vi "minimax.vi"(0 "depth":i32=-1, 1 "redTurn":i32=-1, 2 "mode/difficulty":i32, 5 "mX":i32=-1, 7 "mY":i32=-1, 9 "exist":i32[][](array[numeric])=[[0, 0, 0, 0, 0, 0, 0, 0], [0, 0, 0, 0, 0, 0, 0, 0], [0, 0, 0, 0, 0, 0, 0, 0], [0, 0, 0, 0, 0, 0, 0, 0], [0, 0, 0, 0, 0, 0, 0, 0], [0, 0, 0, 0, 0, 0, 0, 0], [0, 0, 0, 0, 0, 0, 0, 0], [0, 0, 0, 0, 0, 0, 0, 0]], 11 "pos":i32[][](array[numeric])=[[0, 0, 0, 0, 0, 0, 0, 0], [0, 0, 0, 0, 0, 0, 0, 0], [0, 0, 0, 0, 0, 0, 0, 0], [0, 0, 0, 0, 0, 0, 0, 0], [0, 0, 0, 0, 0, 0, 0, 0], [0, 0, 0, 0, 0, 0, 0, 0], [0, 0, 0, 0, 0, 0, 0, 0], [0, 0, 0, 0, 0, 0, 0, 0]], 12 "alpha":i32=-1, 13 "beta":i32=-1) -> (4 "minimax":dbl, 6 "mXnew":i32=-1, 8 "mYnew":i32=-1, 10 "existNew":i32[][](array[numeric]), 15 "posNew":i32[][](array[numeric]))   [LabVIEW 2022 SP3, in "subvis.lvlib"]
uses:
  subvis.lvlib
panel:
  out "j":i32
  out "i":i32
  out "h":dbl
  out "newS.exist":i32[][](array[numeric])
  out "newS.pos":i32[][](array[numeric])
  out "newAvailables":i32[][](array[numeric])
  out "finish":bool
  out "bestHeu":dbl
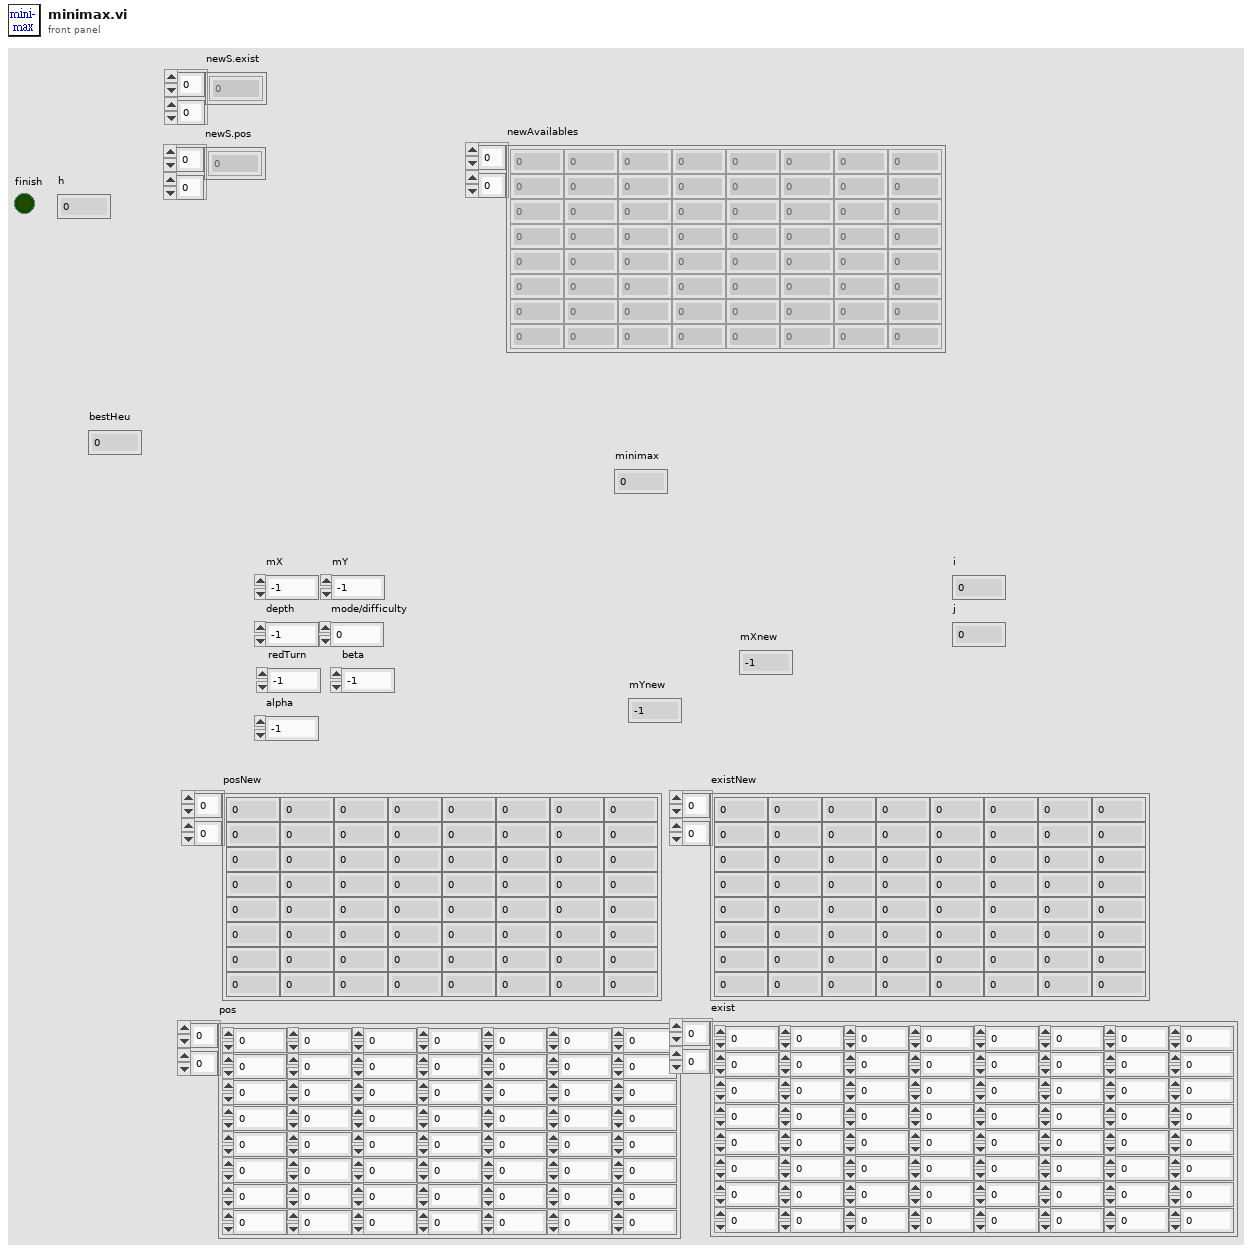
[diagram p1: front panel]
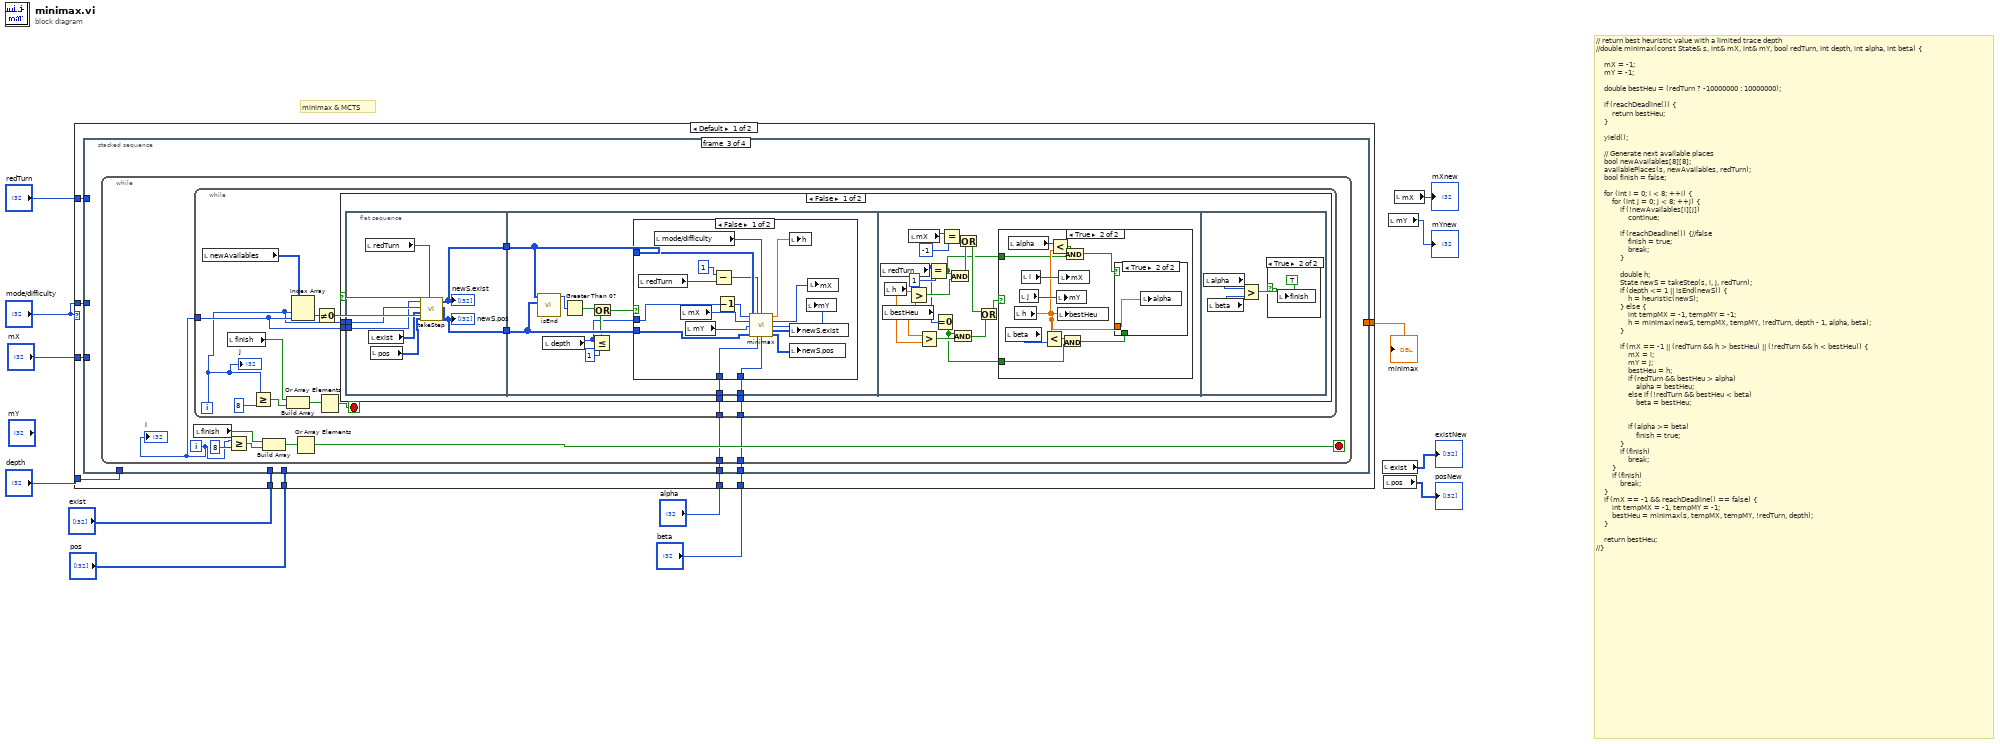
[diagram p0: block diagram]
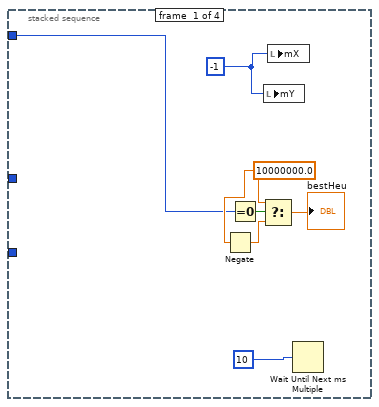
[diagram p2: hidden frame]
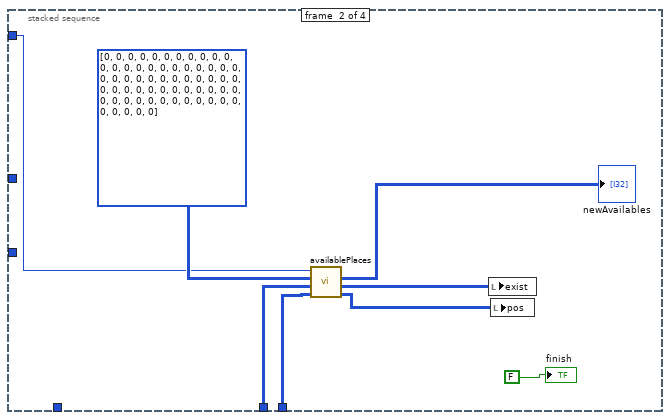
[diagram p3: hidden frame]
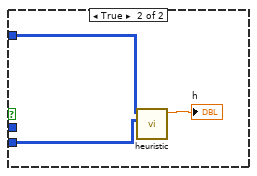
[diagram p4: hidden frame]
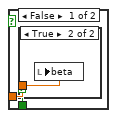
[diagram p6: hidden frame]
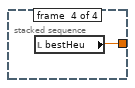
[diagram p10: hidden frame]
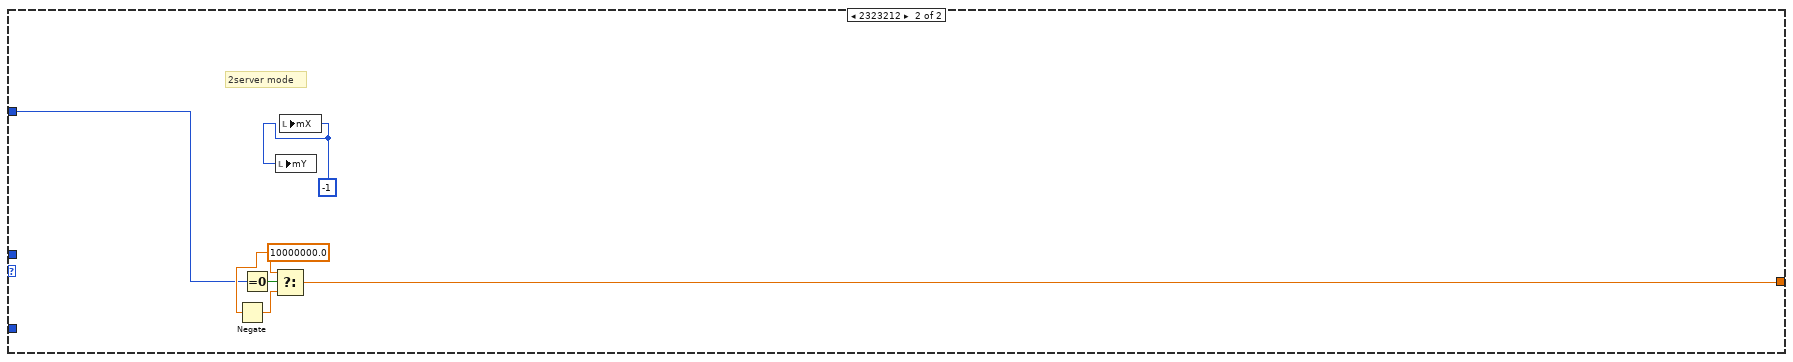
[diagram p11: hidden frame]
diagram:
  # "minimax & MCTS"
  # "// return best heuristic value with a limited trace depth\n//double minimax(const State& s, int& mX, int& mY, bool redTurn, int depth, int alpha, int beta) {\n\n    mX = -1;\n    mY = -1;\n\n    double bestHeu = (redTurn ? -10000000 : 10000000);\n\n    if (reachDeadline()) {\n        return bestHeu;\n    }\n\n    yield();\n\n    // Generate next available places\n    bool newAvailables[8][8];\n    availablePlaces(s, newAvailables, redTurn);\n    bool finish = false;\n\n    for (int i = 0; i < 8; ++i) {\n        for (int j = 0; j < 8; ++j) {\n            if (!newAvailables[i][j])\n                continue;\n\n            if (reachDeadline()) {//false\n                finish = true;\n                break;\n            }\n\n            double h;\n            State newS = takeStep(s, i, j, redTurn);\n            if (depth <= 1 || isEnd(newS)) {\n                h = heuristic(newS);\n            } else {\n                int tempMX = -1, tempMY = -1;\n                h = minimax(newS, tempMX, tempMY, !redTurn, depth - 1, alpha, beta);\n            }\n\n            if (mX == -1 || (redTurn && h > bestHeu) || (!redTurn && h < bestHeu)) {\n                mX = i;\n                mY = j;\n                bestHeu = h;\n                if (redTurn && bestHeu > alpha)\n                    alpha = bestHeu;\n                else if (!redTurn && bestHeu < beta)\n                    beta = bestHeu;\n\n\n                if (alpha >= beta)\n                    finish = true;\n            }\n            if (finish)\n                break;\n        }\n        if (finish)\n            break;\n    }\n    if (mX == -1 && reachDeadline() == false) {\n        int tempMX = -1, tempMY = -1;\n        bestHeu = minimax(s, tempMX, tempMY, !redTurn, depth);\n    }\n\n    return bestHeu;\n//}"
  n1 = case shown="Default" "mode/difficulty" {
    tunnel: [w16 w139] -> w13
    tunnel: "redTurn" -> [w22 w138]
    tunnel: "exist" -> [w21 _]
    tunnel: "pos" -> [w20 _]
    tunnel: "mX" -> [w19 _]
    tunnel: "depth" -> [w18 _]
    tunnel: "mode/difficulty" -> [w17 _]
    tunnel: "alpha" -> [w15 _]
    tunnel: "beta" -> [w14 _]
    frame Default {
      n2 = stacked-sequence {
        tunnel: w22 -> [w23 w30 _ _]
        tunnel: w21 -> [_ w35 _ _]
        tunnel: w20 -> [_ w34 _ _]
        tunnel: w19 -> [_ _ _ _]
        tunnel: w18 -> [_ _ _ _]
        tunnel: w17 -> [_ _ _ _]
        tunnel: [_ _ _ w137] -> w16
        tunnel: w15 -> [_ _ w39 _]
        tunnel: w14 -> [_ _ w38 _]
        frame #0 {
          w27 = 10000000.0 ("t")
          w26 = -1
          n3 = Negate(x=w27) -> (-x=w28:dbl)
          n4 = Equal To 0?(x=w23) -> (x = 0?=w29:bool)
          n5 = Select(t=w27, s=w29, f=w28) -> (s? t:f=→"bestHeu":dbl)
          n6 = local write "mY"(w26) -> ()
          n7 = local write "mX"(w26) -> ()
          n8 = Wait Until Next ms Multiple(millisecond multiple=u32 10) -> ()  [unwired: 1 out]
        }
        frame #1 {
          n9 = call "availablePlaces.vi"("pos"=w34, "exist"=w35, "available"=i32[][] [[0, 0, 0, 0, 0, 0, 0, 0], [0, 0, 0, 0, 0, 0, 0, 0], [0, 0, 0, 0, 0, 0, 0, 0], [0, 0, 0, 0, 0, 0, 0, 0], [0, 0, 0, 0, 0, 0, 0, 0], [0, 0, 0, 0, 0, 0, 0, 0], [0, 0, 0, 0, 0, 0, 0, 0], [0, 0, 0, 0, 0, 0, 0, 0]], "redTurn"=w30) -> ("posNew"=w32:i32[][], "existNew"=w33:i32[][], "availableNew"=→"newAvailables":i32[][])  [unwired: 4 in, 1 out]
          n10 = local write "exist"(w33) -> ()
          n11 = local write "pos"(w32) -> ()
          "finish" <- FALSE
        }
        frame #2 {
          n12 = while {
            tunnel: w39 -> [w41]
            tunnel: w38 -> [w40]
            i -> [w42]
            stop <- w46 stop-if-true
            n13 = local read "finish"() -> (w43:bool)
            n14 = while {
              tunnel: w42 -> [w51]
              tunnel: w41 -> [w49]
              tunnel: w40 -> [w48]
              i -> [w50]
              stop <- w57 stop-if-true
              n15 = local read "newAvailables"() -> (w54:i32[][])
              n16 = local read "finish"() -> (w56:bool)
              n17 = Greater Or Equal?(x=w50, y=8) -> (x >= y?=w55:bool)
              n18 = Build Array(w56, w55) -> (w59:bool[])
              n19 = Index Array(array=w54, index (row)=w50, index (col)=w51) -> (element=w53:i32)
              n20 = Not Equal To 0?(x=w53) -> (x != 0?=w52:bool)
              n21 = Or Array Elements(Boolean array=w59) -> (logical OR=w57:bool)
              n22 = case shown="False" w52 {
                tunnel: w51 -> [w65 _]
                tunnel: w50 -> [w64 _]
                tunnel: w49 -> [w61 _]
                tunnel: w48 -> [w60 _]
                frame False {
                  n23 = flat-sequence {
                    tunnel: w65 -> [w67]
                    tunnel: w64 -> [w68]
                    tunnel: [w72] -> w63
                    tunnel: [w71] -> w62
                    tunnel: w63 -> [w81]
                    tunnel: w62 -> [w80]
                    tunnel: w61 -> [w74]
                    tunnel: w60 -> [w73]
                    frame #0 {
                      n24 = local read "redTurn"() -> (w66:i32)
                      n25 = local read "exist"() -> (w70:i32[][])
                      n26 = local read "pos"() -> (w69:i32[][])
                      n27 = call "takeStep.vi"("redTurn"=w66, "pos"=w69, "exist"=w70, "j"=w68, "i"=w67) -> ("posNew"=w71:i32[][], "existNew"=w72:i32[][])  [unwired: 4 in, 1 out]
                      "newS.exist" <- w72
                      "newS.pos" <- w71
                    }
                    frame #1 {
                      n28 = call "isEnd.vi"("pos"=w80, "exist"=w81) -> ("isEnd"=w82:i16)  [unwired: 9 in]
                      n29 = local read "depth"() -> (w75:i32)
                      n30 = Greater Than 0?(x=w82) -> (x > 0?=w79:bool)
                      n31 = Less Or Equal?(x=w75, y=1) -> (x <= y?=w78:bool)
                      n32 = Or(x=w79, y=w78) -> (x .or. y?=w76:bool)
                      n33 = case shown="False" w76 {
                        tunnel: w81 -> [w98 w102]
                        tunnel: w80 -> [w97 w101]
                        tunnel: w75 -> [w96 _]
                        tunnel: w74 -> [w84 _]
                        tunnel: w73 -> [w83 _]
                        frame False {
                          n34 = local read "redTurn"() -> (w95:i32)
                          n35 = local read "mode/difficulty"() -> (w92:i32)
                          n36 = local read "mX"() -> (w86:i32)
                          n37 = local read "mY"() -> (w85:i32)
                          n38 = Subtract(x=1, y=w95) -> (x-y=w93:i32)
                          n39 = Decrement(x=w96) -> (x-1=w89:i32)
                          n40 = call "minimax.vi"("depth"=w89, "redTurn"=w93, "mode/difficulty"=w92, "mX"=w86, "mY"=w85, "exist"=w98, "pos"=w97, "alpha"=w84, "beta"=w83) -> ("minimax"=w99:dbl, "mXnew"=w88:i32, "mYnew"=w87:i32, "existNew"=w90:i32[][], "posNew"=w91:i32[][])  [unwired: 2 in]
                          n41 = local write "h"(w99) -> ()
                          n42 = local write "newS.exist"(w90) -> ()
                          n43 = local write "newS.pos"(w91) -> ()
                          n44 = local write "mY"(w87) -> ()
                          n45 = local write "mX"(w88) -> ()
                        }
                        frame True {
                          n46 = call "heuristic.vi"("pos"=w101, "exist"=w102) -> ("heuristic"=→"h":dbl)  [unwired: 9 in]
                        }
                      }
                    }
                    frame #2 {
                      n47 = local read "redTurn"() -> (w109:i32)
                      n48 = local read "bestHeu"() -> (w108:dbl)
                      n49 = local read "h"() -> (w107:dbl)
                      n50 = Greater?(x=w107, y=w108) -> (0:w110:bool)
                      n51 = local read "mX"() -> (w117:i32)
                      n52 = Greater?(x=w108, y=w107) -> (0:w106:bool)
                      n53 = Equal?(x=w109, y=1) -> (x = y?=w104:bool)
                      n54 = Equal To 0?(x=w109) -> (x = 0?=w103:bool)
                      n55 = Equal?(x=w117, y=-1) -> (x = y?=w115:bool)
                      n56 = And(x=w104, y=w110) -> (x .and. y?=w113:bool)
                      n57 = And(x=w103, y=w106) -> (x .and. y?=w112:bool)
                      n58 = Or(x=w115, y=w113) -> (x .or. y?=w114:bool)
                      n59 = Or(x=w114, y=w112) -> (x .or. y?=w105:bool)
                      n60 = case shown="True" w105 {
                        tunnel: w104 -> [_ w118]
                        tunnel: w103 -> [_ w120]
                        frame False {
                        }
                        frame True {
                          n61 = local read "beta"() -> (w123:i32)
                          n62 = local read "alpha"() -> (w125:i32)
                          n63 = local read "h"() -> (w122:dbl)
                          n64 = local read "j"() -> (w127:i32)
                          n65 = local read "i"() -> (w128:i32)
                          n66 = Less?(x=w122, y=w123) -> (x < y?=w121:bool)
                          n67 = Less?(x=w125, y=w122) -> (x < y?=w126:bool)
                          n68 = local write "mY"(w127) -> ()
                          n69 = local write "bestHeu"(w122) -> ()
                          n70 = local write "mX"(w128) -> ()
                          n71 = And(x=w121, y=w120) -> (x .and. y?=w119:bool)
                          n72 = And(x=w126, y=w118) -> (x .and. y?=w124:bool)
                          n73 = case shown="True" w124 {
                            tunnel: w122 -> [w130 w132]
                            tunnel: w119 -> [w129 _]
                            frame False {
                              n74 = case shown="True" w129 {
                                tunnel: w130 -> [_ w131]
                                frame False {
                                }
                                frame True {
                                n75 = local write "beta"(w131) -> ()
                                }
                              }
                            }
                            frame True {
                              n76 = local write "alpha"(w132) -> ()
                            }
                          }
                        }
                      }
                    }
                    frame #3 {
                      n77 = local read "alpha"() -> (w133:i32)
                      n78 = local read "beta"() -> (w134:i32)
                      n79 = Greater?(x=w133, y=w134) -> (0:w135:bool)
                      n80 = case shown="True" w135 {
                        frame False {
                        }
                        frame True {
                          n81 = local write "finish"(TRUE ("finish")) -> ()
                        }
                      }
                    }
                  }
                }
                frame True {
                }
              }
              "j" <- w50
            }
            n82 = Greater Or Equal?(x=w42, y=8) -> (x >= y?=w45:bool)
            n83 = Build Array(w43, w45) -> (w44:bool[])
            n84 = Or Array Elements(Boolean array=w44) -> (logical OR=w46:bool)
            "i" <- w42
          }
        }
        frame #3 {
          n85 = local read "bestHeu"() -> (w137:dbl)
        }
      }
    }
    frame 2323212 {
      w141 = 10000000.0 ("t")
      w140 = -1
      # "2server mode"
      n86 = Negate(x=w141) -> (-x=w142:dbl)
      n87 = Equal To 0?(x=w138) -> (x = 0?=w143:bool)
      n88 = Select(t=w141, s=w143, f=w142) -> (s? t:f=w139:dbl)
      n89 = local write "mY"(w140) -> ()
      n90 = local write "mX"(w140) -> ()
    }
  }
  "minimax" <- w13
  n91 = local read "exist"() -> (→"existNew":i32[][])
  n92 = local read "pos"() -> (→"posNew":i32[][])
  n93 = local read "mY"() -> (→"mYnew":i32)
  n94 = local read "mX"() -> (→"mXnew":i32)
